vi "SendDatabase2Cerebus.vi"(1 "Database":T1={"ExperimentDate"=timestamp(3401556199.892892 s since 1904-01-01), "ImplantDate"=timestamp(3401890063 s since 1904-01-01), "CerebusFolder"="", "Experimenter"="Tyler Davis", "NHPName"="201102", "DeviceType"="uECOG", "DeviceSerial"="CG-64BPX-F419", "DeviceHemisphere"="Right", "DeviceRegion"="Hand", "TaskType"="ArmMovementTask.vi", "TaskComments"="", "RecordingComments"="", "GeneralObservations"=""}) -> (0 "ParameterString":string)   [LabVIEW 2013]
panel:
  # "Do not place ';' or '=' in the comment fields"
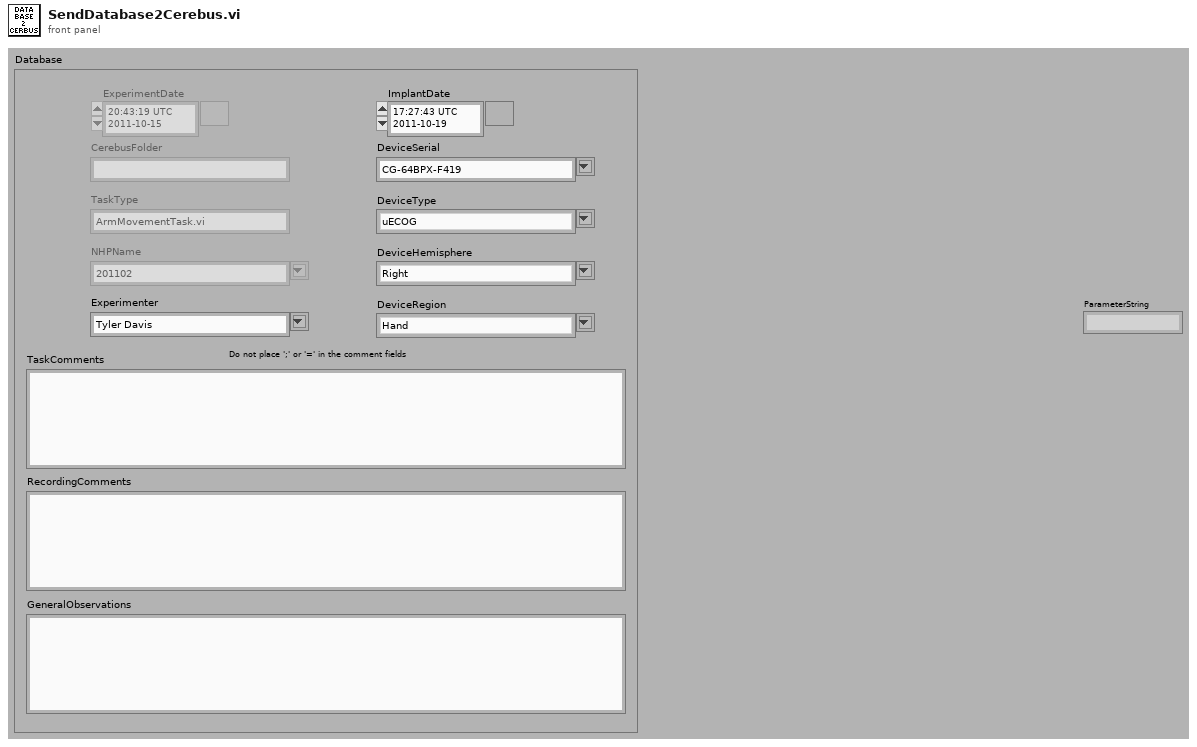
[diagram p1: front panel]
types:
  T1 = cluster{"ExperimentDate":timestamp, "ImplantDate":timestamp, "CerebusFolder":string, "Experimenter":string, "NHPName":string, "DeviceType":string, "DeviceSerial":string, "DeviceHemisphere":string, "DeviceRegion":string, "TaskType":string, "TaskComments":string, "RecordingComments":string, "GeneralObservations":string}
  T2 = enum16{"Initialize", "String", "Start", "New Session", "Stop", "Resume", "Close"}
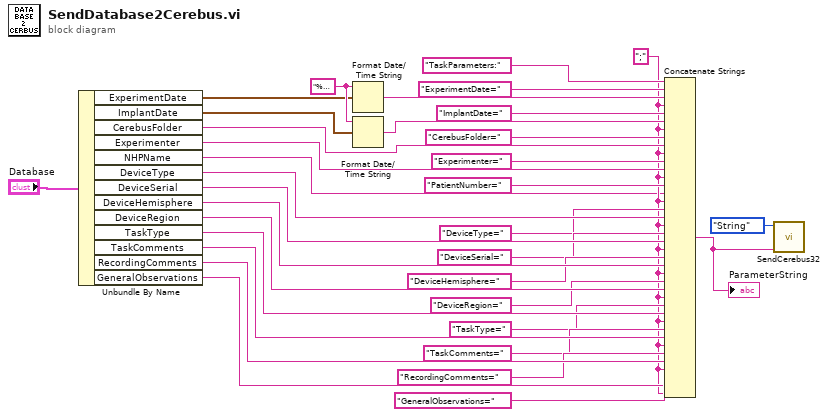
[diagram p0: block diagram]
diagram:
  w5 = ";" ("element")
  w11 = "%Y%m%d-%H%M%S" ("time format string (%c)")
  n1 = Unbundle By Name("Database") -> ("ExperimentDate"=w9:timestamp, "ImplantDate"=w10:timestamp, "CerebusFolder"=w26:string, "Experimenter"=w27:string, "NHPName"=w1:string, "DeviceType"=w28:string, "DeviceSerial"=w29:string, "DeviceHemisphere"=w30:string, "DeviceRegion"=w31:string, "TaskType"=w32:string, "TaskComments"=w33:string, "RecordingComments"=w34:string, "GeneralObservations"=w6:string)
  n2 = Format Date/Time String(time format string (%c)=w11, seconds (now)=w9) -> (date/time string=w24:string)  [unwired: 1 in]
  n3 = Format Date/Time String(time format string (%c)=w11, seconds (now)=w10) -> (date/time string=w25:string)  [unwired: 1 in]
  n4 = Concatenate Strings("TaskParameters:" ("string"), "ExperimentDate=" ("string"), w24, w5, "ImplantDate=" ("string"), w25, w5, "CerebusFolder=" ("string"), w26, w5, "Experimenter=" ("string"), w27, w5, "PatientNumber=" ("string"), w1, w5, "DeviceType=" ("string"), w28, w5, "DeviceSerial=" ("string"), w29, w5, "DeviceHemisphere=" ("string"), w30, w5, "DeviceRegion=" ("string"), w31, w5, "TaskType=" ("string"), w32, w5, "TaskComments=" ("string"), w33, w5, "RecordingComments=" ("string"), w34, w5, "GeneralObservations=" ("string"), w6, w5) -> (w3:string)
  "ParameterString" <- w3
  n5 = call "SendCerebus32.vi"("String"=w3, "Mode"=T2."String") -> ()  [unwired: 3 in]
